vi "Abort Sequence.vi"() -> ()   [LabVIEW 2022 SP3]
uses:
  RT Controls/DO FGV.ctl
panel:
  out "DO out":bool[](array[boolean])
  in  "DI 2":T1(array[cluster])=[{"CDT"=-150.0, "Position"=TRUE, "Component ID"="F_EPV_131", "Con(T)-Cum(F)"=FALSE, "No.of.Sam"=0.0, "Abort File"="", "Duration"=0}, {"CDT"=-150.0, "Position"=TRUE, "Component ID"="F_EPV_131", "Con(T)-Cum(F)"=FALSE, "No.of.Sam"=0.0, "Abort File"="", "Duration"=0}, {"CDT"=-135.0, "Position"=FALSE, "Component ID"="F_EPV_132", "Con(T)-Cum(F)"=FALSE, "No.of.Sam"=0.0, "Abort File"="", "Duration"=0}, {"CDT"=-120.0, "Position"=FALSE, "Component ID"="F_EPV_131", "Con(T)-Cum(F)"=FALSE, "No.of.Sam"=0.0, "Abort File"="", "Duration"=0}, {"CDT"=-20.0, "Position"=TRUE, "Component ID"="F_EPV_136", "Con(T)-Cum(F)"=FALSE, "No.of.Sam"=0.0, "Abort File"="", "Duration"=0}, {"CDT"=-10.0, "Position"=FALSE, "Component ID"="F_EPV_136", "Con(T)-Cum(F)"=FALSE, "No.of.Sam"=0.0, "Abort File"="", "Duration"=0}]
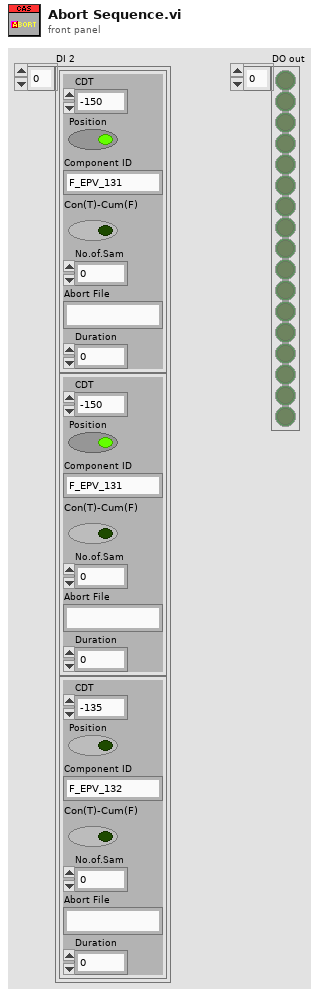
[diagram p1: front panel]
types:
  T1 = cluster{"CDT":dbl, "Position":bool, "Component ID":string, "Con(T)-Cum(F)":bool, "No.of.Sam":dbl, "Abort File":string, "Duration":u32}[]
  T2 = typedef "DO FGV.ctl" = enum16{"Read", "Write", "Start time", "init", "Read only"}
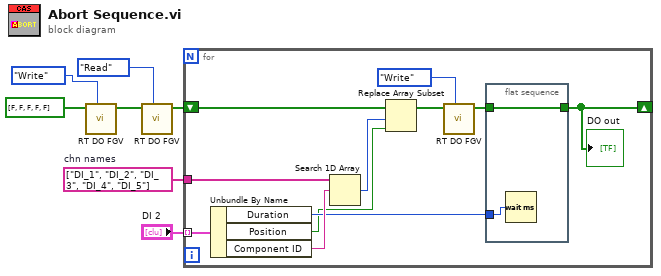
[diagram p0: block diagram]
diagram:
  w6 = string[] ["DI_1", "DI_2", "DI_3", "DI_4", "DI_5"]  # chn names
  n1 = call "RT DO FGV.vi"("Enum"=DO_FGV."Write", "DO in"=bool[] [FALSE, FALSE, FALSE, FALSE, FALSE]) -> ("DO out"=w1:bool[])  [unwired: 7 in, 2 out]
  n2 = call "RT DO FGV.vi"("Enum"=DO_FGV."Read", "DO in"=w1) -> ("DO out"=w4:bool[])  [unwired: 7 in, 2 out]
  n3 = for {
    tunnel: "DI 2" -> [w18] mode=indexing
    tunnel: w6 -> [w16]
    shift-right: [w8] -> _
    shift-left: w4 -> [w13]
    n4 = Unbundle By Name(w18) -> ("Duration"=w14:u32, "Position"=w11:bool, "Component ID"=w15:string)
    n5 = Search 1D Array(1D array=w16, element=w15) -> (index of element=w12:i32)  [unwired: 1 in]
    n6 = Replace Array Subset(array=w13, new element=w11, index=w12) -> (w10:bool[])
    n7 = call "RT DO FGV.vi"("Enum"=DO_FGV."Write", "DO in"=w10) -> ("DO out"=w9:bool[])  [unwired: 7 in, 2 out]
    n8 = flat-sequence {
      tunnel: w14 -> [w20]
      tunnel: w9 -> [w19]
      tunnel: [w19] -> w8
      frame #0 {
        n9 = Wait (ms)(milliseconds to wait=w20) -> ()  [unwired: 1 out]
      }
    }
    "DO out" <- w8
  }
